vi "UPortal Load Calendar.vi"(6 "timeout (50000)":i32=50000, 8 "error in":errorcluster, 11 "Calendar URL":string="https://users.magnet.fsu.edu/Experiments/Calendar.aspx") -> (0 "error out":errorcluster, 3 "Events out":T1[](array[typedef]))   [LabVIEW 2020]
uses:
  Utilities/iCalendar/Extract iCalendar String.ctl
  <vilib>/httpClient/LabVIEWHTTPClient.lvlib
panel:
  out "body":string
  out "headers":string
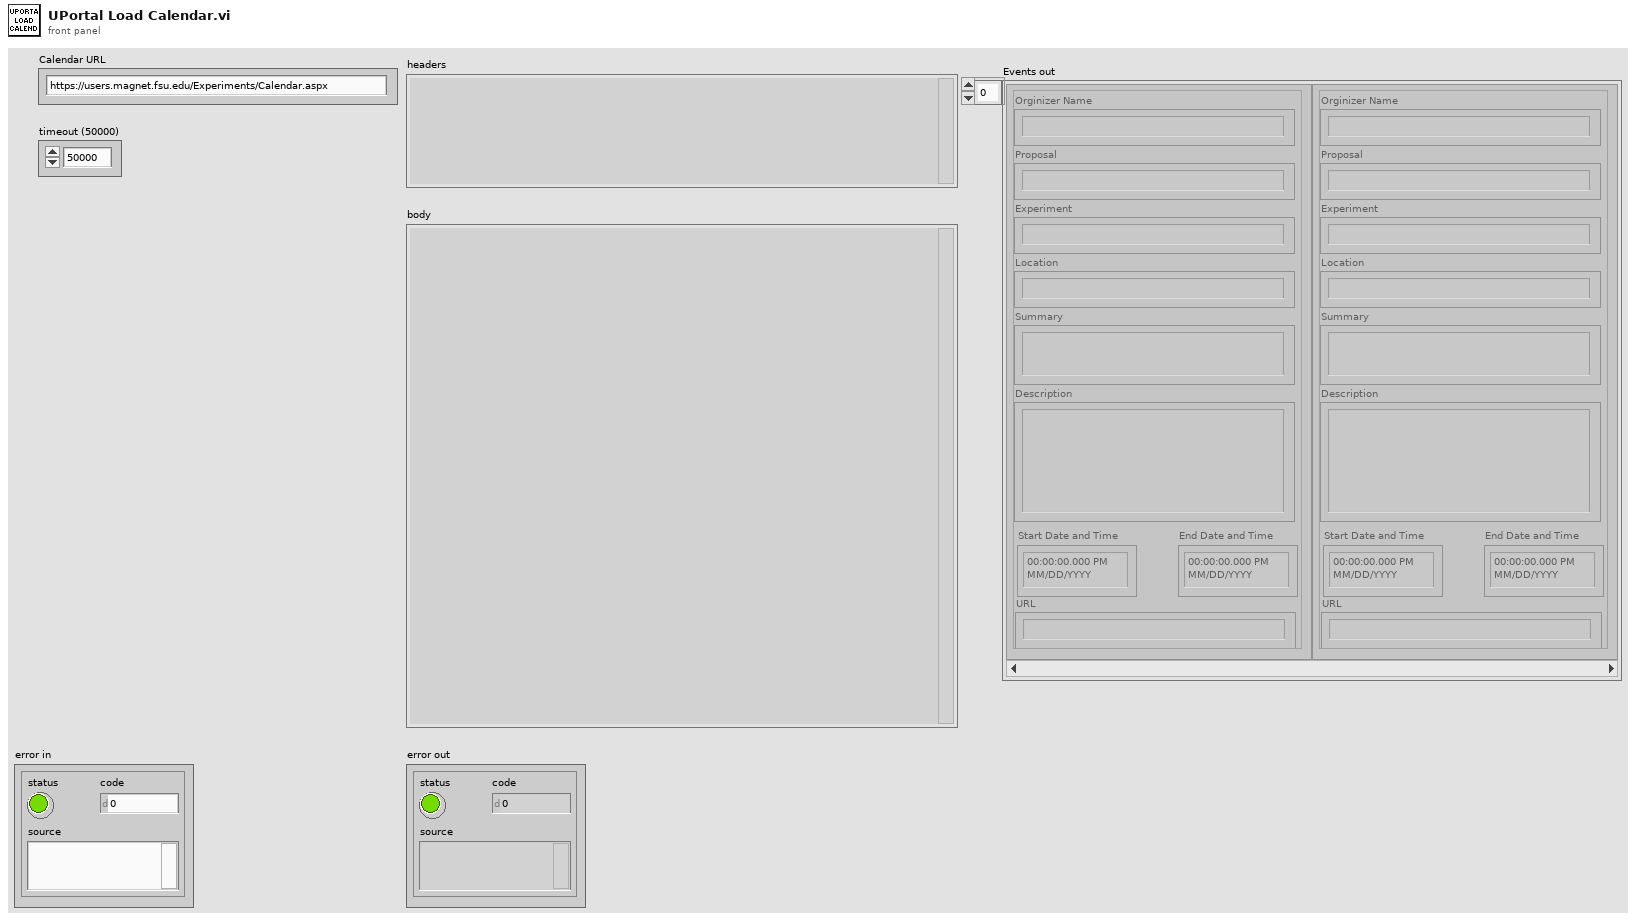
[diagram p1: front panel]
types:
  T1 = typedef "Extract iCalendar String.ctl" = cluster{"Orginizer Name":string, "Location":string, "Summary":string, "Start Date and Time":timestamp, "End Date and Time":timestamp, "Description":string, "Proposal":string, "Experiment":string, "URL":string}
  T2 = typedef "LabVIEWHTTPClient.lvlib/ClientHandle.ctl" = refnum<k1>
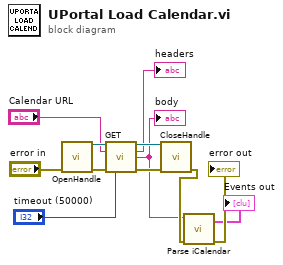
[diagram p0: block diagram]
diagram:
  n1 = call <vilib>:"OpenHandle.vi"("error in (no error)"="error in") -> ("client handle out"=w11:T2, "error out"=w10:errorcluster)  [unwired: 13 in]
  n2 = call <vilib>:"GET.vi"("client handle"=w11, "url"="Calendar URL", "error in (no error)"=w10, "timeout (10000)"="timeout (50000)") -> ("client handle out"=w7:T2, "headers"=→"headers":string, "body"=w2:string, "error out"=w8:errorcluster)  [unwired: 8 in]
  "body" <- w2
  n3 = call <vilib>:"CloseHandle.vi"("client handle"=w7, "error in (no error)"=w8) -> ("error out"=w4:errorcluster)  [unwired: 13 in]
  n4 = call "Parse iCalendar.vi"("error in"=w4, "iCalendar string"=w2) -> ("error out"=→"error out":errorcluster, "Events out"=→"Events out":T1[])  [unwired: 7 in, 1 out]
